vi "Delete.vi"(8 "Error In":errorcluster, 11 "QwtPlotItem in":refnum<class "QwtPlotItem.lvclass">) -> (0 "Error Out":errorcluster)   [LabVIEW 2014, in "QwtPlotItem.lvclass"]
doc: "This dynamic dispatch VI is intended to free the memory that was allocated to this object. Override this VI to property deallocate your subclass if necessary.\n\nThe default implementation does not delete anything, but produces an warning."
uses:
  QwtPlotItem.lvclass
  LQ Core/LQIdentity/LQIdentity.lvclass/LQIdentity.ctl
  LQ Core/LQCoreEngine/_Internal/LQIdentity Registry Action.ctl
  LQ Core/LQIdentity/LQIdentity.lvclass
  LQ Core/LQ Core.lvlib
  LQ Core/LQCoreEngine/LQCoreEngine.lvclass
panel:
  # "Copyright (c) 2021 Sze Howe Koh\n\nThis Source Code Form is subject to the terms of the Mozilla Public\nLicense, v. 2.0. If a copy of the MPL was not distributed with this\nfile, You can obtain one at http://mozilla.org/MPL/2.0/."
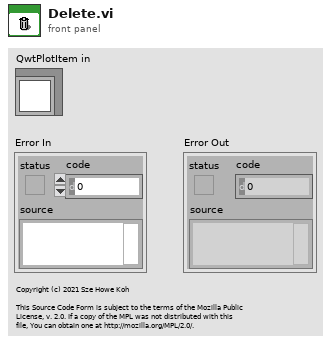
[diagram p1: front panel]
types:
  T1 = typedef "LQ Core.lvlib/LQCoreEngine.lvclass/LQIdentity Registry Action.ctl" = enum16{"Init", "Register LQIdentity", "Get LQIdentity Info", "Deregister LQIdentity"}
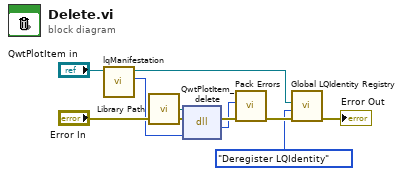
[diagram p0: block diagram]
diagram:
  n1 = call "lqManifestation.vi"("LQIdentity in"="QwtPlotItem in") -> ("Manifestation"=w8:u64, "LQIdentity out"=w4:refnum<class "QwtPlotItem.lvclass">)  [unwired: 9 in]
  n2 = call "Library Path.vi"() -> ("Library Path"=w9:path)
  n3 = dll-call lib="?" fn="QwtPlotItem_delete"(path in=w9, error in="Error In", "_instance"=w8) -> (error out=w7:errorcluster, "errorCode"=w6:i32)  [unwired: 2 in, 1 out]
  n4 = call "Pack Errors.vi"("Error In"=w7, "Error Code"=w6) -> ("Error Out"=w5:errorcluster)  [unwired: 9 in]
  n5 = call "Global LQIdentity Registry.vi"("Error In"=w5, "Registry Action"=LQIdentity_Registry_Action."Deregister LQIdentity", "LQIdentity Info In"=w4) -> ("Error Out"=→"Error Out":errorcluster)  [unwired: 7 in, 1 out]
